vi "Save Config.vi"(8 "error in (no error)":errorcluster, 11 "ConfigAPI in":refnum<class "ConfigAPI.lvclass">) -> (0 "error out":errorcluster, 3 "ConfigAPI out":refnum<class "ConfigAPI.lvclass">)   [LabVIEW 2020, in "Volatus.lvlib" / "ConfigAPI.lvclass"]
uses:
  ConfigAPI.lvclass
  ConfigAPI.lvclass/ConfigAPI.ctl
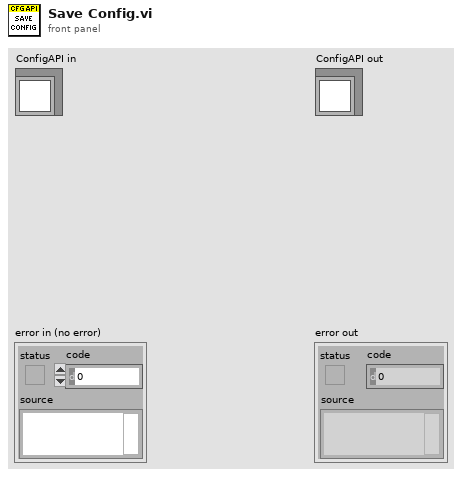
[diagram p1: front panel]
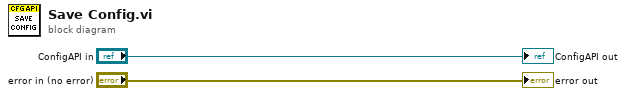
[diagram p0: block diagram]
diagram:
  "error out" <- "error in (no error)"
  "ConfigAPI out" <- "ConfigAPI in"
